vi "SynapseAPI-Get Block.vi"(0 "URL":string="http://localhost:24414", 11 "error in (no error)":errorcluster) -> (8 "block":string, 15 "error out":errorcluster)   [LabVIEW 2020]
uses:
  <vilib>/httpClient/LabVIEWHTTPClient.lvlib
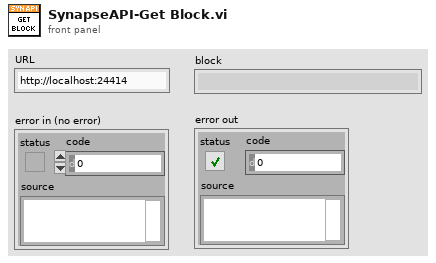
[diagram p1: front panel]
types:
  T1 = typedef "LabVIEWHTTPClient.lvlib/ClientHandle.ctl" = refnum<k1>
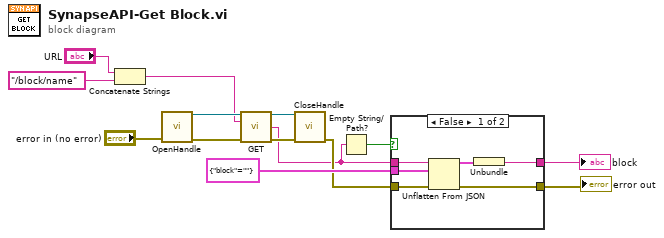
[diagram p0: block diagram]
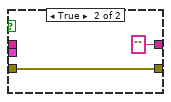
[diagram p2: hidden frame]
diagram:
  n1 = Concatenate Strings("URL", "/block/name") -> (w8:string)
  n2 = call <vilib>:"OpenHandle.vi"("error in (no error)"="error in (no error)") -> ("client handle out"=w11:T1, "error out"=w10:errorcluster)  [unwired: 13 in]
  n3 = call <vilib>:"GET.vi"("client handle"=w11, "url"=w8, "error in (no error)"=w10) -> ("client handle out"=w13:T1, "body"=w2:string, "error out"=w14:errorcluster)  [unwired: 9 in, 1 out]
  n4 = call <vilib>:"CloseHandle.vi"("client handle"=w13, "error in (no error)"=w14) -> ("error out"=w5:errorcluster)  [unwired: 13 in]
  n5 = Empty String/Path?(string/path=w2) -> (empty?=w1:bool)
  n6 = case shown="False" w1 {
    tunnel: w2 -> [w20 _]
    tunnel: cluster{"block":string} {"block"=""} ("Cluster") -> [w19 _]
    tunnel: [w18 w22] -> w6
    tunnel: w5 -> [w17 w22]
    tunnel: [w15 "" ("block")] -> w3
    frame False {
      n7 = Unflatten From JSON(JSON string=w20, type and defaults=w19, error in (no error)=w17) -> (value=w16:cluster{"block":string}, error out=w18:errorcluster)  [unwired: 4 in]
      n8 = Unbundle(w16) -> ("block"=w15:string)
    }
    frame True {
    }
  }
  "error out" <- w6
  "block" <- w3
